vi "z_StringGetThrough_.vi"(8 "Error In":errorcluster, 9 "String In":string) -> (0 "Error Out":errorcluster, 1 "String Out":string)   [LabVIEW 2012]
doc: "This device shifts a sstring through.\nIt can be used to pass a string to a variable within an error chain. For example a status message can be updated at a certain location."
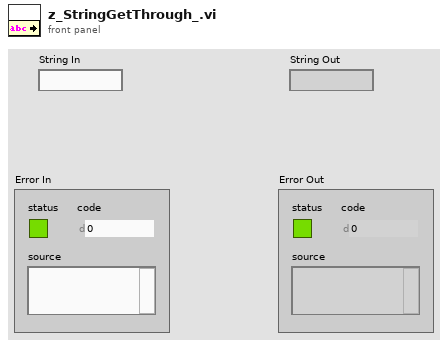
[diagram p1: front panel]
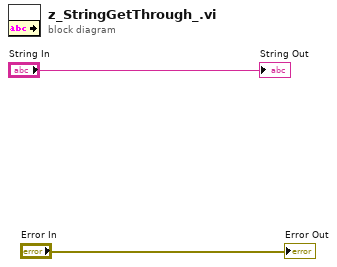
[diagram p0: block diagram]
diagram:
  "Error Out" <- "Error In"
  "String Out" <- "String In"
